vi "DIGIT_5122_Stop_Session.vi"(8 "error in (no error)":errorcluster, 11 "instrument handle":refnum<k15> caption="instrument handle in") -> (0 "error out":errorcluster)   [LabVIEW 2017]
doc: "Aborts an acquisition even if the digitizer times out waiting for a trigger. \nCloses the instrument I/O session. \nDeallocates any memory resources used by the IVI session."
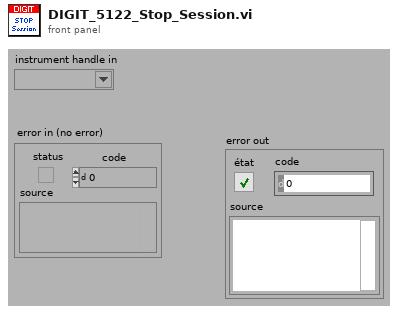
[diagram p1: front panel]
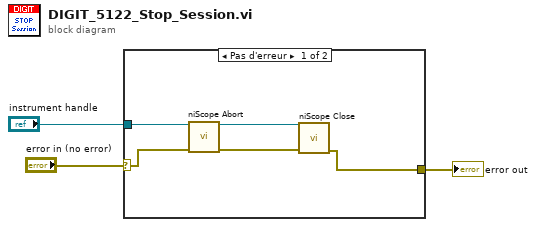
[diagram p0: block diagram]
diagram:
  n1 = case shown="Pas d'erreur" "error in (no error)" {
    selector: "error in (no error)" -> [w5 w9]
    tunnel: [w4 w9] -> w3
    tunnel: "instrument handle" -> [w6 _]
    frame No Error {
      n2 = call <instrlib>:"niScope Abort.vi"("instrument handle"=w6, "error in"=w5) -> ("instrument handle out"=w7:refnum<k15>, "error out"=w8:errorcluster)  [unwired: 12 in]
      n3 = call <instrlib>:"niScope Close.vi"("instrument handle"=w7, "error in"=w8) -> ("error out"=w4:errorcluster)  [unwired: 13 in]
    }
    frame Error {
    }
  }
  "error out" <- w3
